vi "S2C_PCIe1762H_Proc_PortCount.vi"(8 "Error In":errorcluster) -> (0 "Error Out":errorcluster, 3 "Result":string)   [LabVIEW 2024]
uses:
  S2C_PCIe1762H_Proc_Globals.vi
  <userlib>/DAQNavi Polymorphic VI/create/DAQNavi Create Channel(DO-Digital Output).vi
  <userlib>/DAQNavi Polymorphic VI/configure/DAQNavi Get Property/DO/DAQNaviGet_DO_PortCount.vi
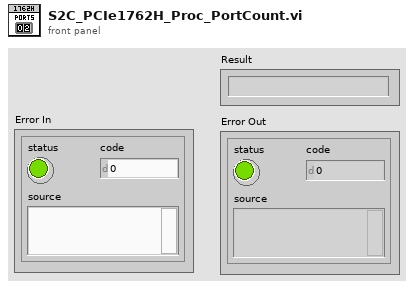
[diagram p1: front panel]
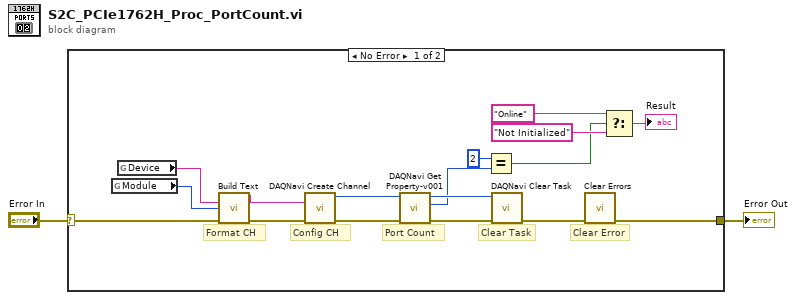
[diagram p0: block diagram]
diagram:
  n1 = case shown="No Error" "Error In" {
    selector: "Error In" -> [w5 w20]
    tunnel: [w4 w20] -> w1
    frame No Error {
      # "Clear Error"
      # "Clear Task"
      # "Port Count"
      # "Format CH"
      # "Config CH"
      n2 = global read "S2C_PCIe1762H_Proc_Globals.vi" "Module"() -> (w12:i32)
      n3 = global read "S2C_PCIe1762H_Proc_Globals.vi" "Device"() -> (w11:string)
      n4 = call "Build Text"("Device"=w11, "Module"=w12, "error in (no error)"=w5) -> ("Result"=w3:string, "error out"=w19:errorcluster)  [unwired: 11 in]
      n5 = call-poly <userlib>:"DAQNavi Create Channel.vi"("physical channels"=w3, "error in (no error)"=w19) -> ("task out"=w9:i32, "error out"=w10:errorcluster)  [unwired: 3 in, 9 out]
      n6 = call-poly <userlib>:"DAQNavi Get Property-v001.vi"("error in (no error)"=w10, "task in"=w9) -> ("error out"=w18:errorcluster, "port count"=w8:i32, "task out"=w17:i32)  [unwired: 7 in]
      n7 = Equal?(x=2, y=w8) -> (x = y?=w6:bool)
      n8 = call <userlib>:"DAQNavi Clear Task.vi"("error in (no error)"=w18, "task in"=w17) -> ("error out"=w13:errorcluster)  [unwired: 1 out]
      n9 = call <vilib>:"Clear Errors.vi"("error in (no error)"=w13) -> ("error out"=w4:errorcluster)  [unwired: 5 in, 1 out]
      n10 = Select(t="Online", s=w6, f="Not Initialized") -> (s? t:f=→"Result":string)
    }
    frame Error {
    }
  }
  "Error Out" <- w1
